vi "Untitled 1.vi"() -> ()   [LabVIEW 2010]
panel:
  out "1 2":dbl
  in  "1":dbl
  in  "OK Button":bool
  in  "stop":bool
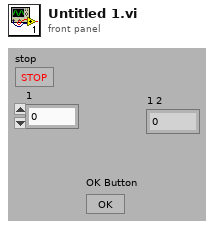
[diagram p1: front panel]
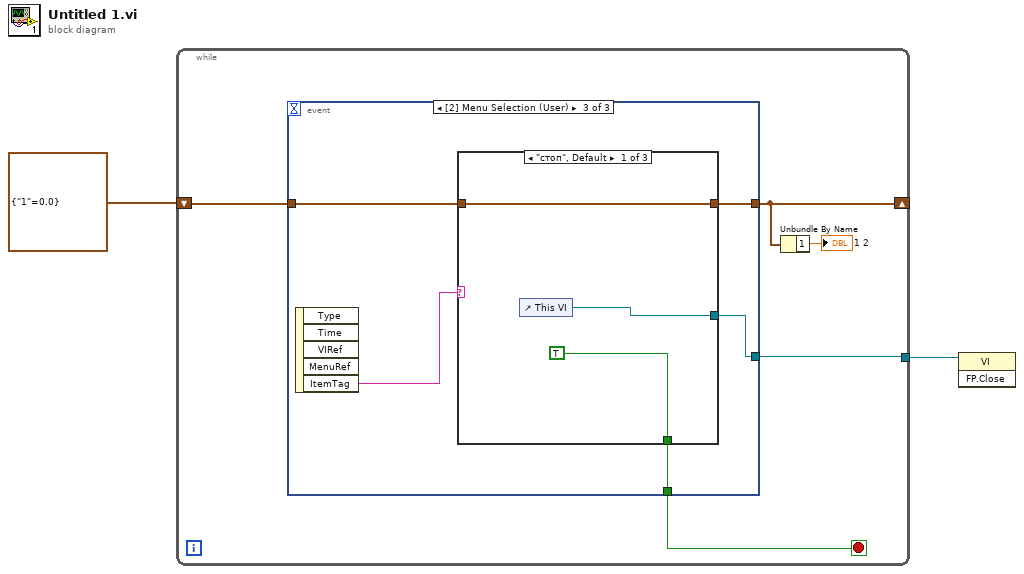
[diagram p0: block diagram]
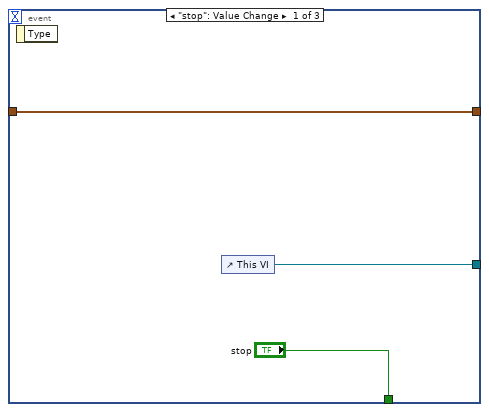
[diagram p2: hidden frame]
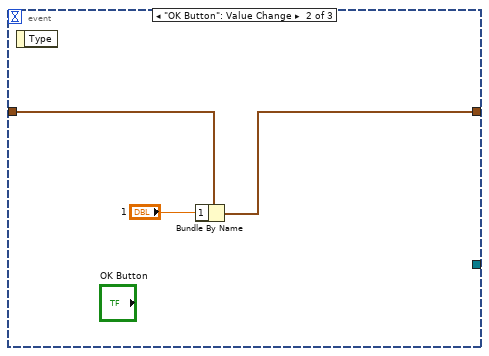
[diagram p3: hidden frame]
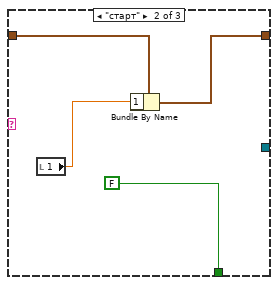
[diagram p4: hidden frame]
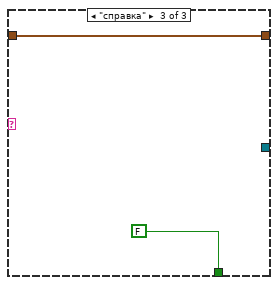
[diagram p5: hidden frame]
diagram:
  n1 = while {
    shift-right: [w5] -> _
    shift-left: cluster{"1":dbl} {"1"=0.0} -> [w6]
    tunnel: [w3] -> w1
    stop <- w7 stop-if-true
    n2 = event shown="[2] Menu Selection (User)" {
      selector: _ -> [_ _ _]
      dyn-events: _ -> [_ _ _]
      timeout: _ -> [_ _ _]
      tunnel: ["stop" _ w17] -> w7
      tunnel: w6 -> [w9 w13 w16]
      tunnel: [w9 w12 w15] -> w5
      tunnel: [w8 _ w14] -> w3
      event "stop": Value Change {
        n3 = event-data() -> ()  [unwired: 1 in, 1 out]
        n4 = control-ref of="This VI"() -> (w8:refnum<vi>)
      }
      event "OK Button": Value Change {
        n5 = event-data() -> ()  [unwired: 1 in, 1 out]
        n6 = Bundle By Name(cluster=w13, "1"="1") -> (w12:cluster{"1":dbl})
      }
      event Menu Selection (User) {
        n7 = event-data() -> ("ItemTag"=w18:string)  [unwired: 1 in, 4 out]
        n8 = case shown="\"стоп\", Default" w18 {
          tunnel: [TRUE FALSE FALSE] -> w17
          tunnel: w16 -> [w20 w25 w27]
          tunnel: [w20 w24 w27] -> w15
          tunnel: [w19 _ _] -> w14
          frame "стоп", Default {
            n9 = control-ref of="This VI"() -> (w19:refnum<vi>)
          }
          frame "старт" {
            n10 = local read "1"() -> (w23:dbl)
            n11 = Bundle By Name(cluster=w25, "1"=w23) -> (w24:cluster{"1":dbl})
          }
          frame "справка" {
          }
        }
      }
    }
    n12 = Unbundle By Name(w5) -> ("1"=→"1 2":dbl)
  }
  n13 = invoke class="VI" method="FP.Close"(reference=w1) -> ()  [unwired: 2 in, 3 out]
